vi "测试状态判断.vi"(10 "配置信息":T9={"周期模式"=enum."不启用", "测量参数"={"氨氮"=TRUE, "总磷"=TRUE, "总氮"=TRUE, "CODMn"=TRUE, "CODCr"=FALSE}, "定点周期"={"启动命令"=enum."", "启动命令 2"=enum."", "启动命令 3"=enum."", "启动命令 4"=enum."", "启动命令 5"=enum."", "启动命令 6"=enum."", "启动命令 7"=enum."", "启动命令 8"=enum."", "启动命令 9"=enum."", "启动命令 10"=enum."", "启动命令 11"=enum."", "启动命令 12"=enum."", "启动命令 13"=enum."", "启动命令 14"=enum."", "启动命令 15"=enum."", "启动命令 16"=enum."", "启动命令 17"=enum."", "启动命令 18"=enum."", "启动命令 19"=enum."", "启动命令 20"=enum."", "启动命令 21"=enum."", "启动命令 22"=enum."", "启动命令 23"=enum."", "启动命令 24"=enum.""}, "间隔启动"={"启动命令"=enum."", "启动间隔"=0.0, "启动次数"=0}}, 11 "Display State In":T1={"仪器状态"=FALSE, "仪器时间"=timestamp(0 s since 1904-01-01), "测量参数"={"氨氮"=TRUE, "总磷"=TRUE, "总氮"=TRUE, "CODMn"=TRUE, "CODCr"=FALSE}, "调用模块名称"="", "测试状态"={"启动时间"=timestamp(0 s since 1904-01-01), "结束时间"=timestamp(0 s since 1904-01-01), "启动次数"=0.0}}) -> (1 "Data In":T3={"启动"=FALSE, "控制命令"=enum."加标回收（启动采配水）", "测量参数"={"氨氮"=TRUE, "总磷"=TRUE, "总氮"=TRUE, "CODMn"=TRUE, "CODCr"=FALSE}} caption="数据", 2 "配置信息读取":T9={"周期模式"=enum."不启用", "测量参数"={"氨氮"=TRUE, "总磷"=TRUE, "总氮"=TRUE, "CODMn"=TRUE, "CODCr"=FALSE}, "定点周期"={"启动命令"=enum."", "启动命令 2"=enum."", "启动命令 3"=enum."", "启动命令 4"=enum."", "启动命令 5"=enum."", "启动命令 6"=enum."", "启动命令 7"=enum."", "启动命令 8"=enum."", "启动命令 9"=enum."", "启动命令 10"=enum."", "启动命令 11"=enum."", "启动命令 12"=enum."", "启动命令 13"=enum."", "启动命令 14"=enum."", "启动命令 15"=enum."", "启动命令 16"=enum."", "启动命令 17"=enum."", "启动命令 18"=enum."", "启动命令 19"=enum."", "启动命令 20"=enum."", "启动命令 21"=enum."", "启动命令 22"=enum."", "启动命令 23"=enum."", "启动命令 24"=enum.""}, "间隔启动"={"启动命令"=enum."", "启动间隔"=0.0, "启动次数"=0}}, 3 "Display State Out":T1={"仪器状态"=FALSE, "仪器时间"=timestamp(0 s since 1904-01-01), "测量参数"={"氨氮"=TRUE, "总磷"=TRUE, "总氮"=TRUE, "CODMn"=TRUE, "CODCr"=FALSE}, "调用模块名称"="", "测试状态"={"启动时间"=timestamp(0 s since 1904-01-01), "结束时间"=timestamp(0 s since 1904-01-01), "启动次数"=0.0}})   [LabVIEW 2016, in "ZK定时设置.xctl"]
uses:
  <vilib>/ptbypt/NI_PtbyPt.lvlib
panel:
  # "分钟"
  # "次"
  # "分钟"
  # "次"
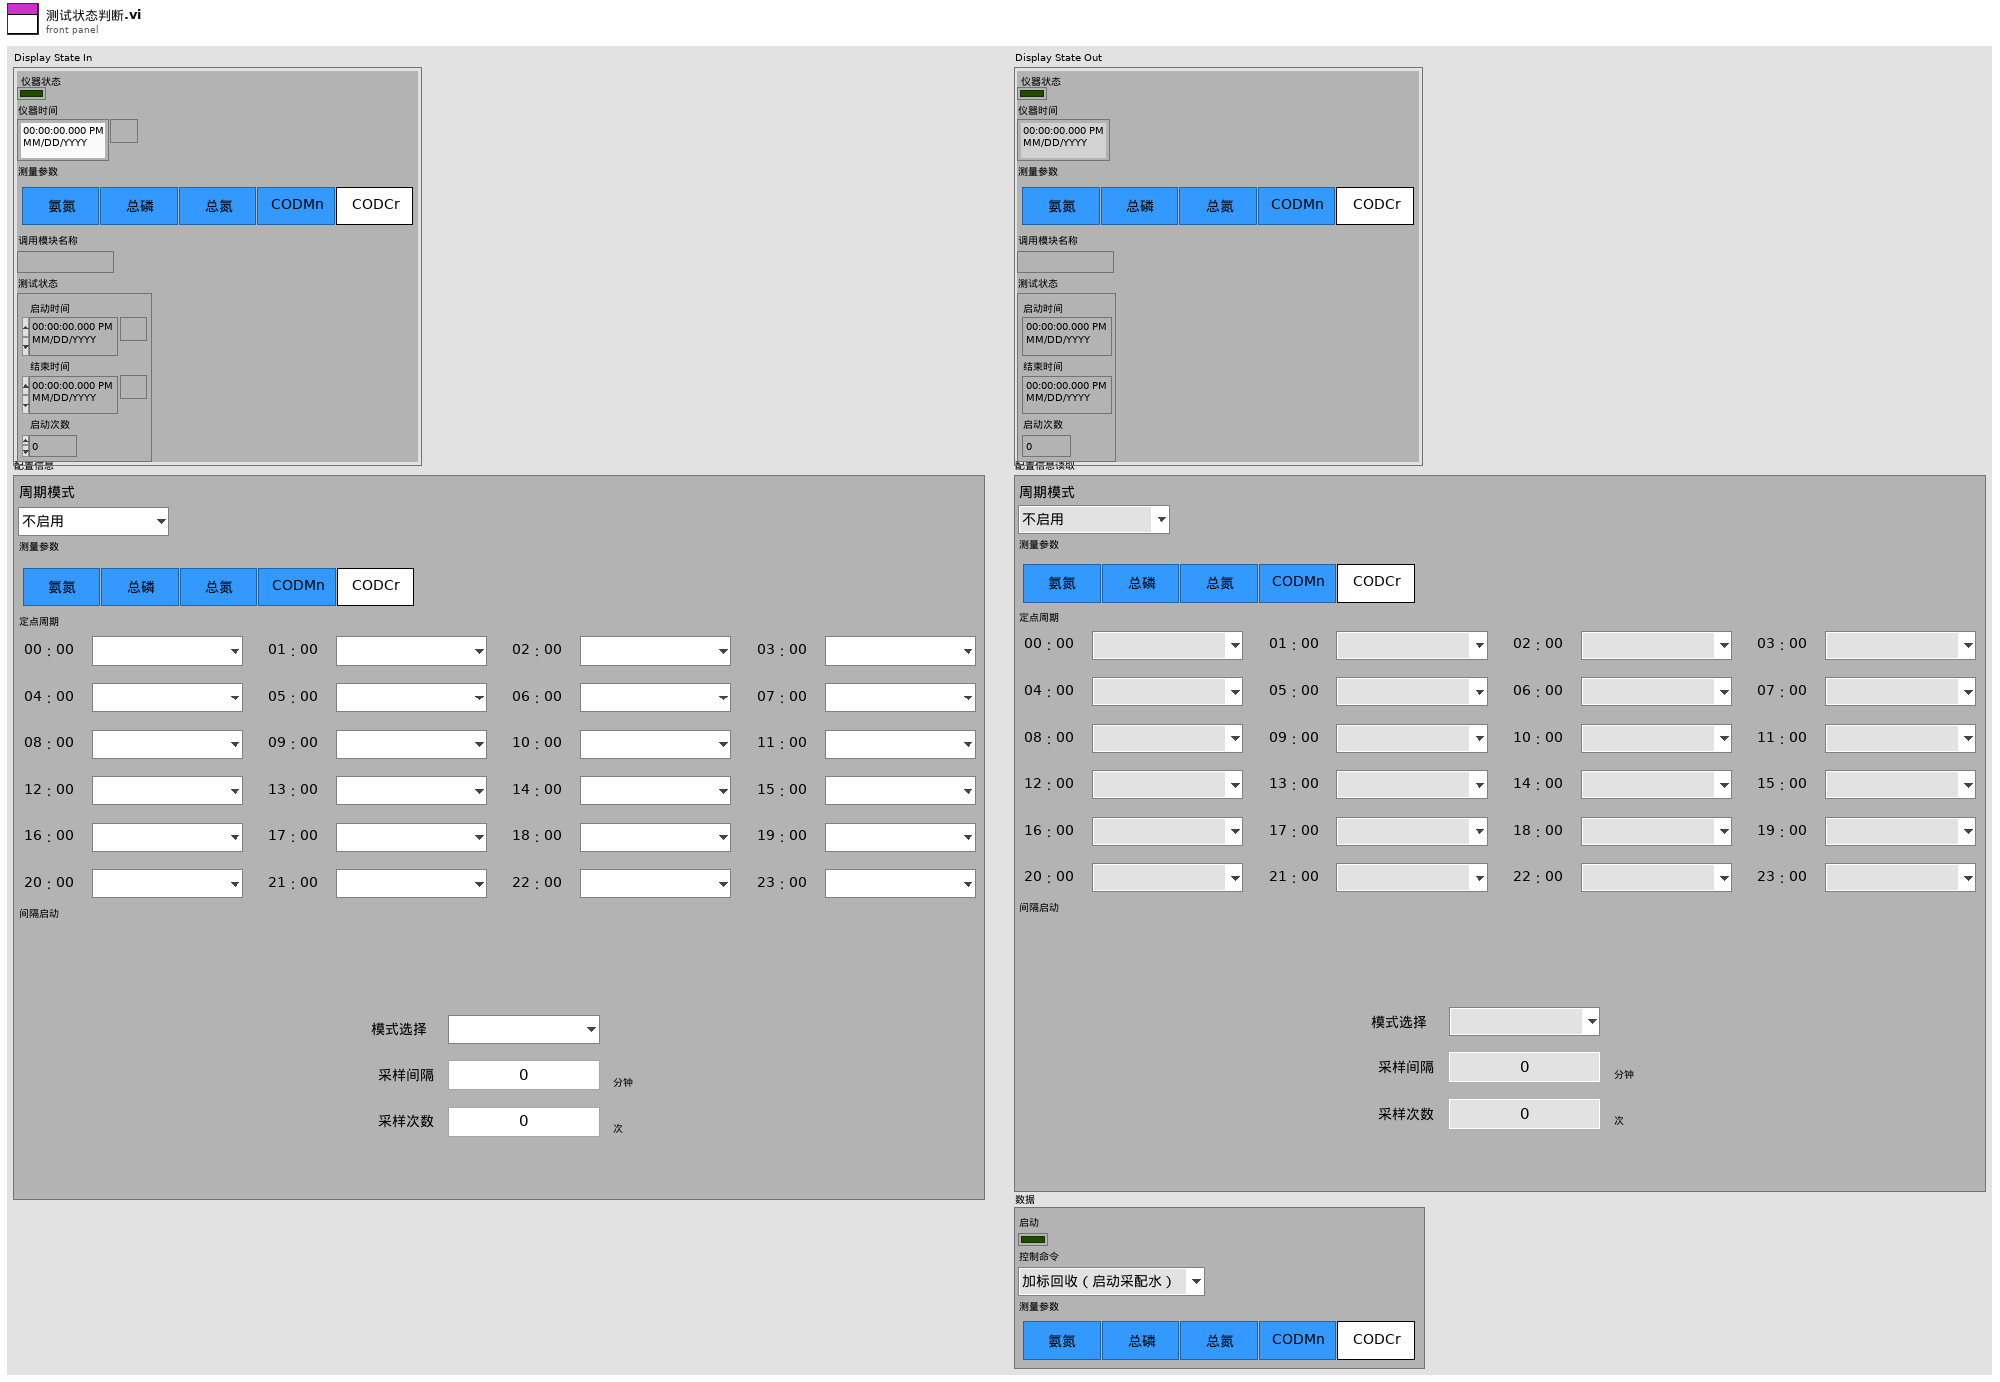
[diagram p1: front panel]
types:
  T1 = typedef "ZK定时设置.xctl/状态 1.ctl" = cluster{"仪器状态":bool, "仪器时间":timestamp, "测量参数":T2, "调用模块名称":string, "测试状态":cluster{"启动时间":timestamp, "结束时间":timestamp, "启动次数":dbl}}
  T2 = typedef "ZK定时设置.xctl/测量参数.ctl" = cluster{"氨氮":bool, "总磷":bool, "总氮":bool, "CODMn":bool, "CODCr":bool}
  T3 = typedef "ZK定时设置.xctl/数据 1.ctl" = cluster{"启动":bool, "控制命令":T4, "测量参数":T2}
  T4 = typedef "ZK定时设置.xctl/国标控制命令.ctl" = enum16{"加标回收（启动采配水）", "加标回收（不启动采配水）", "水样测试（启动采配水）", "水样测试（不启动采配水）", "平行样测试（启动采配水）", "平行样测试（不启动采配水）", "集成干预测试"}
  T5 = typedef "ZK定时设置.xctl/周期模式设置.ctl" = enum16{"不启用", "定点模式", "间隔模式"}
  T6 = typedef "ZK定时设置.xctl/定点周期设置.ctl" = cluster{"启动命令":T7, "启动命令 2":T7, "启动命令 3":T7, "启动命令 4":T7, "启动命令 5":T7, "启动命令 6":T7, "启动命令 7":T7, "启动命令 8":T7, "启动命令 9":T7, "启动命令 10":T7, "启动命令 11":T7, "启动命令 12":T7, "启动命令 13":T7, "启动命令 14":T7, "启动命令 15":T7, "启动命令 16":T7, "启动命令 17":T7, "启动命令 18":T7, "启动命令 19":T7, "启动命令 20":T7, "启动命令 21":T7, "启动命令 22":T7, "启动命令 23":T7, "启动命令 24":T7}
  T7 = typedef "ZK定时设置.xctl/启动命令选择.ctl" = enum16{"", "加标回收（启动采配水）", "加标回收（不启动采配水）", "水样测试（启动采配水）", "水样测试（不启动采配水）", "平行样测试（启动采配水）", "平行样测试（不启动采配水）", "集成干预测试"}
  T8 = typedef "ZK定时设置.xctl/间隔启动设置.ctl" = cluster{"启动命令":T7, "启动间隔":dbl, "启动次数":i32}
  T9 = cluster{"周期模式":T5, "测量参数":T2, "定点周期":T6, "间隔启动":T8}
  T10 = cluster{"启动时间":timestamp, "结束时间":timestamp, "启动次数":dbl}
  T11 = typedef "LVDateTimeRec.ctl" = cluster{"秒数的小数部分":dbl, "秒":i32, "分":i32, "时":i32, "日":i32, "月":i32, "年":i32, "天数（周）":i32, "天数（年）":i32, "DST":i32}
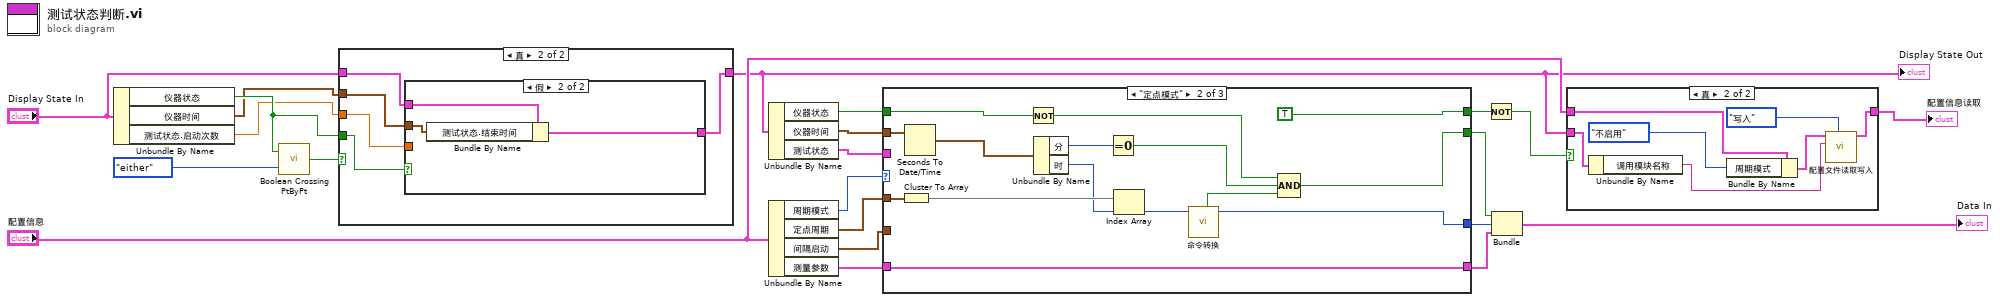
[diagram p0: block diagram]
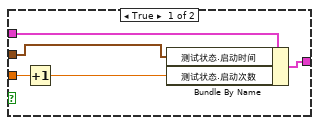
[diagram p4: hidden frame]
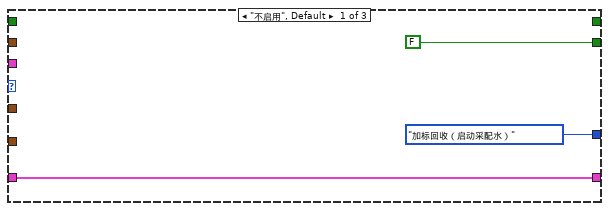
[diagram p5: hidden frame]
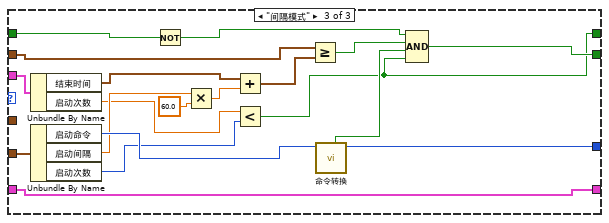
[diagram p6: hidden frame]
diagram:
  n1 = Unbundle By Name("Display State In") -> ("仪器状态"=w11:bool, "仪器时间"=w6:timestamp, "测试状态.启动次数"=w5:dbl)
  n2 = call <vilib>:"Boolean Crossing PtByPt.vi"("direction"=enum16{"either", "false-true", "true-false"}."either", "input"=w11) -> ("crossing"=w12:bool)  [unwired: 1 in]
  n3 = case shown="真" w12 {
    tunnel: "Display State In" -> [w23 w26]
    tunnel: [w23 w28] -> w2
    tunnel: w11 -> [_ w27]
    tunnel: w6 -> [_ w25]
    tunnel: w5 -> [_ w24]
    frame False {
    }
    frame True {
      n4 = case shown="假" w27 {
        tunnel: w26 -> [w31 w36]
        tunnel: w25 -> [w33 w35]
        tunnel: [w32 w34] -> w28
        tunnel: w24 -> [w29 _]
        frame True {
          n5 = Increment(x=w29) -> (x+1=w30:dbl)
          n6 = Bundle By Name(cluster=w31, "测试状态.启动时间"=w33, "测试状态.启动次数"=w30) -> (w32:T1)
        }
        frame False {
          n7 = Bundle By Name(cluster=w36, "测试状态.结束时间"=w35) -> (w34:T1)
        }
      }
    }
  }
  "Display State Out" <- w2
  n8 = Unbundle By Name(w2) -> ("仪器状态"=w7:bool, "仪器时间"=w8:timestamp, "测试状态"=w9:T10)
  n9 = Unbundle By Name("配置信息") -> ("周期模式"=w22:T5, "定点周期"=w20:T6, "间隔启动"=w19:T8, "测量参数"=w18:T2)
  n10 = case shown="\"定点模式\"" w22 {
    tunnel: w20 -> [_ w44 _]
    tunnel: w19 -> [_ _ w66]
    tunnel: w8 -> [_ w54 w59]
    tunnel: w7 -> [_ w51 w73]
    tunnel: w18 -> [w37 w47 w69]
    tunnel: [国标控制命令."加标回收（启动采配水）" ("控制命令") w45 w67] -> w16
    tunnel: [FALSE w48 w70] -> w17
    tunnel: [w37 w47 w69] -> w15
    tunnel: w9 -> [_ _ w65]
    tunnel: [_ TRUE w55] -> w3
    frame "不启用", Default {
    }
    frame "定点模式" {
      n11 = Cluster To Array(cluster=w44) -> (array=w43:T7[])
      n12 = Seconds To Date/Time(time stamp (now)=w54) -> (date time rec=w53:T11)  [unwired: 1 in]
      n13 = Not(x=w51) -> (.not. x?=w50:bool)
      n14 = Unbundle By Name(w53) -> ("分"=w52:i32, "时"=w42:i32)
      n15 = Equal To 0?(x=w52) -> (x = 0?=w49:bool)
      n16 = Index Array(array=w43, index=w42) -> (element=w41:T7)
      n17 = call "命令转换.vi"("启动命令"=w41) -> ("控制命令"=w45:T4, "布尔"=w46:bool)  [unwired: 9 in]
      n18 = Compound Arithmetic op=AND ("复合运算")(w50, w49, w46) -> (w48:bool)
    }
    frame "间隔模式" {
      n19 = Unbundle By Name(w65) -> ("结束时间"=w64:timestamp, "启动次数"=w57:dbl)
      n20 = Unbundle By Name(w66) -> ("启动命令"=w71:T7, "启动间隔"=w63:dbl, "启动次数"=w56:i32)
      n21 = Not(x=w73) -> (.not. x?=w72:bool)
      n22 = Multiply(x=w63, y=60.0) -> (x*y=w61:dbl)
      n23 = Add(x=w64, y=w61) -> (x+y=w60:timestamp)
      n24 = Less?(x=w57, y=w56) -> (x < y?=w55:bool)
      n25 = Greater Or Equal?(x=w59, y=w60) -> (x >= y?=w58:bool)
      n26 = call "命令转换.vi"("启动命令"=w71) -> ("控制命令"=w67:T4, "布尔"=w68:bool)  [unwired: 9 in]
      n27 = Compound Arithmetic op=AND ("复合运算")(w72, w58, w68, w55) -> (w70:bool)
    }
  }
  n28 = Not(x=w3) -> (.not. x?=w1:bool)
  n29 = Bundle(w17, "控制命令"=w16, "测量参数"=w15) -> (→"Data In":cluster{bool, "控制命令":T4, "测量参数":T2})  [unwired: 1 in]
  n30 = case shown="真" w1 {
    tunnel: "配置信息" -> [w74 w81]
    tunnel: [w74 w78] -> w4
    tunnel: w2 -> [_ w76]
    frame False {
    }
    frame True {
      n31 = Unbundle By Name(w76) -> ("调用模块名称"=w75:string)
      n32 = Bundle By Name(cluster=w81, "周期模式"=周期模式设置."不启用") -> (w79:T9)
      n33 = call "配置文件读取写入.vi"("配置模式"=enum16{"读取", "写入"}."写入", "配置文件名"=w75, "配置信息"=w79) -> ("配置信息读取"=w78:T9)  [unwired: 7 in, 1 out]
    }
  }
  "配置信息读取" <- w4
